vi "Umgebung.WriteZustandsgrössen.vi"(0 "Umgebung in":refnum<data-value>, 1 "Manuelle Eingabe On/Off":bool, 2 "Sekunden":dbl, 3 "Aussentemperatur [°C] Manuell":dbl, 4 "Solare Gewinne [W] Manuell":dbl, 5 "Error in":errorcluster) -> (19 "Error out":errorcluster)   [LabVIEW 2016, in "Umgebung.lvclass"]
uses:
  Umgebung.lvclass
  Umgebung.lvclass/Umgebung.ctl
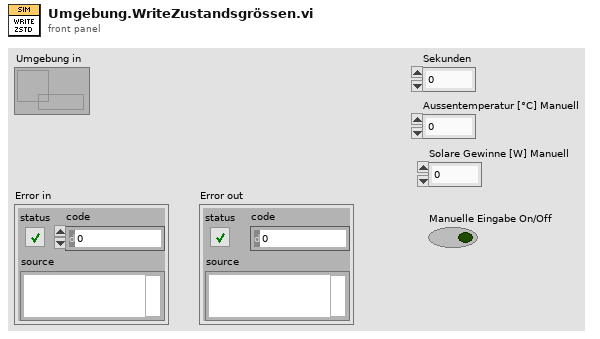
[diagram p1: front panel]
types:
  T1 = typedef "Umgebung.lvclass/Umgebung.Zustandsgrössen.ctl" = cluster{"Aussentemperatur [°C]":dbl, "Aussentemperatur [°C] Manuell":dbl, "Tag":dbl, "Stunde":dbl, "Minute":dbl, "Sekunden":dbl, "Strahlungsleistung [W/m2]":dbl, "Solare Gewinne [W/m2]":dbl, "Solare Gewinne [W/m2] Manuell":dbl, "Manuelle Eingabe On/Off":bool}
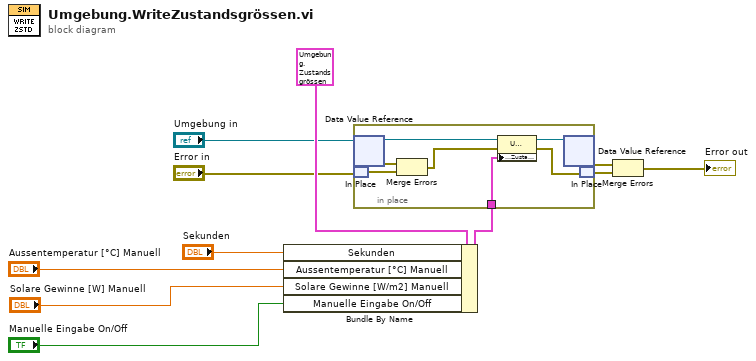
[diagram p0: block diagram]
diagram:
  n1 = Bundle By Name(cluster=T1 {"Aussentemperatur [°C]"=0.0, "Aussentemperatur [°C] Manuell"=0.0, "Tag"=0.0, "Stunde"=0.0, "Minute"=0.0, "Sekunden"=0.0, "Strahlungsleistung [W/m2]"=0.0, "Solare Gewinne [W/m2]"=0.0, "Solare Gewinne [W/m2] Manuell"=0.0, "Manuelle Eingabe On/Off"=FALSE} ("Umgebung.Zustandsgrössen"), "Sekunden"="Sekunden", "Aussentemperatur [°C] Manuell"="Aussentemperatur [°C] Manuell", "Solare Gewinne [W/m2] Manuell"="Solare Gewinne [W] Manuell", "Manuelle Eingabe On/Off"="Manuelle Eingabe On/Off") -> (w7:T1)
  n2 = in-place {
    in-place-border: w7 -> [w12]
    n3 = in-place-dvr #1("Umgebung in") -> (w18:refnum<class "Umgebung.lvclass">, w15:errorcluster)
    n4 = in-place-match #2("Error in") -> (w14:errorcluster)
    n5 = Merge Errors(w15, w14) -> (w16:errorcluster)
    n6 = property class="Umgebung.lvclass"(reference=w18, error in=w16, "Accessors:Umgebung.Zustandsgrössen"=w12) -> (reference out=w17:refnum<class "Umgebung.lvclass">, error out=w13:errorcluster)
    n7 = in-place-dvr #1(w17) -> (w10:errorcluster)  [unwired: 1 out]
    n8 = in-place-match #2(w13) -> (w9:errorcluster)
  }
  n9 = Merge Errors(w10, w9) -> (→"Error out":errorcluster)
